vi "log context.vi"(10 "level":u32(ring) items=["APDM_LL_ALL", "APDM_LL_DEBUG", "APDM_LL_INFO", "APDM_LL_WARNING", "APDM_LL_ERROR", "APDM_LL_NONE"], 11 "context":u32) -> (2 "function return":i32, 3 "context out":u32)   [LabVIEW 2019, in "apdm.lvlib"]
doc: "APDM_EXPORT int apdm_log_context(apdm_ctx_t context, const enum APDM_Logging_Level level);"
uses:
  apdm.lvlib
  Lee Lab/CP FES Walking 2018/Code/Working/LabVIEW/apdm.dll
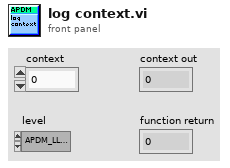
[diagram p1: front panel]
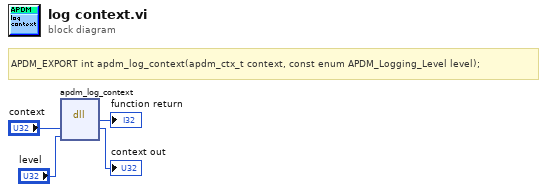
[diagram p0: block diagram]
diagram:
  # "APDM_EXPORT int apdm_log_context(apdm_ctx_t context, const enum APDM_Logging_Level level);"
  n1 = dll-call lib="C:/Users/jfalesi/Dropbox/Lee Lab/CP FES Walking 2018/Code/Working/LabVIEW/apdm.*" fn="apdm_log_context"("context"="context", "level"="level") -> (→"function return":i32, "context"=→"context out":u32)  [unwired: 4 in, 2 out]
